vi "calcDemandedSteps_ToBeDeleted.vi"(8 "error in (no error)":errorcluster, 11 "Model in":refnum<class "Model.lvclass">) -> (0 "error out":errorcluster, 3 "Model out":refnum<class "Model.lvclass">)   [LabVIEW 2015]
uses:
  <userlib>/Common/Devices/StepperMotor/StepperMotor/StepperMotor.lvclass
  <userlib>/Common/ILC/ILC/ILC.lvclass
  Model.lvclass
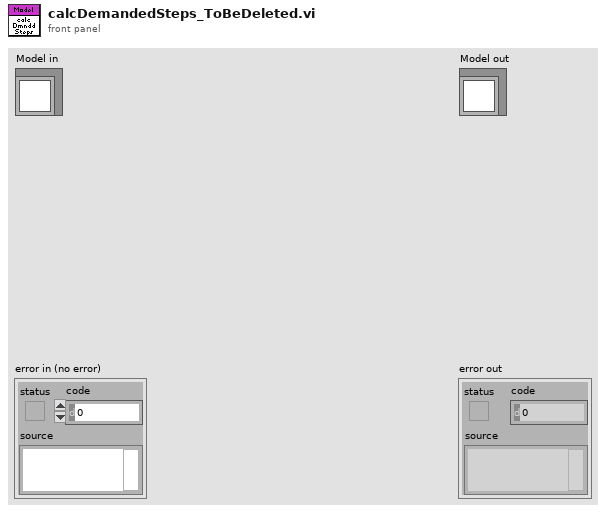
[diagram p1: front panel]
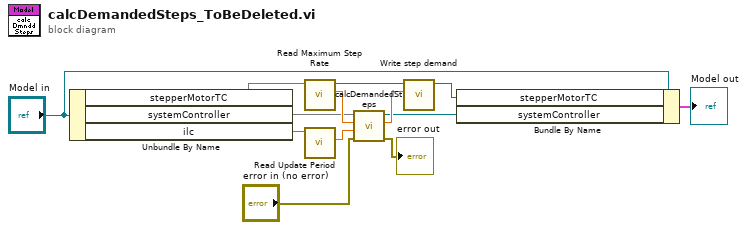
[diagram p0: block diagram]
diagram:
  n1 = Unbundle By Name("Model in") -> ("stepperMotorTC"=w12, "systemController"=w4, "ilc"=w2)
  n2 = call <userlib>:"Read Maximum Step Rate.vi"("StepperMotor in"=w12) -> ("Maximum Step Rate"=w13:dbl[unit], "StepperMotor out"=w11:refnum<class "StepperMotor.lvclass">)  [unwired: 9 in]
  n3 = call <userlib>:"Read Update Period.vi"("ILC in"=w2) -> ("Update Period"=w1:dbl[unit])  [unwired: 9 in, 1 out]
  n4 = call "calcDemandedSteps.vi"("error in (no error)"="error in (no error)", "loopPeriod"=w1, "step rate limit (mag)"=w13, "SystemController in"=w4) -> ("error out"=→"error out":errorcluster, "step demand"=w7:dbl, "SystemController out"=w3:refnum<class "SystemController.lvclass">)  [unwired: 5 in]
  n5 = call <userlib>:"Write step demand.vi"("step demand"=w7, "StepperMotor in"=w11) -> ("StepperMotor out"=w8:refnum<class "StepperMotor.lvclass">)  [unwired: 9 in]
  n6 = Bundle By Name(cluster="Model in", "stepperMotorTC"=w8, "systemController"=w3) -> (→"Model out":cluster{})
